vi "cubeSubstraction.vi"() -> ()   [LabVIEW 2016]
panel:
  out "size(s) 3":i32[](array[numeric])
  out "processed cube 2":i32[][](graph)
  out "reference":i32[][](graph)
  out "processed cube":i32[][](graph)
  out "raw cube":i32[][](graph)
  out "size(s)":i32[](array[numeric])
  out "size(s) 2":i32[](array[numeric])
  out "x-y":i32[][][](array[numeric])
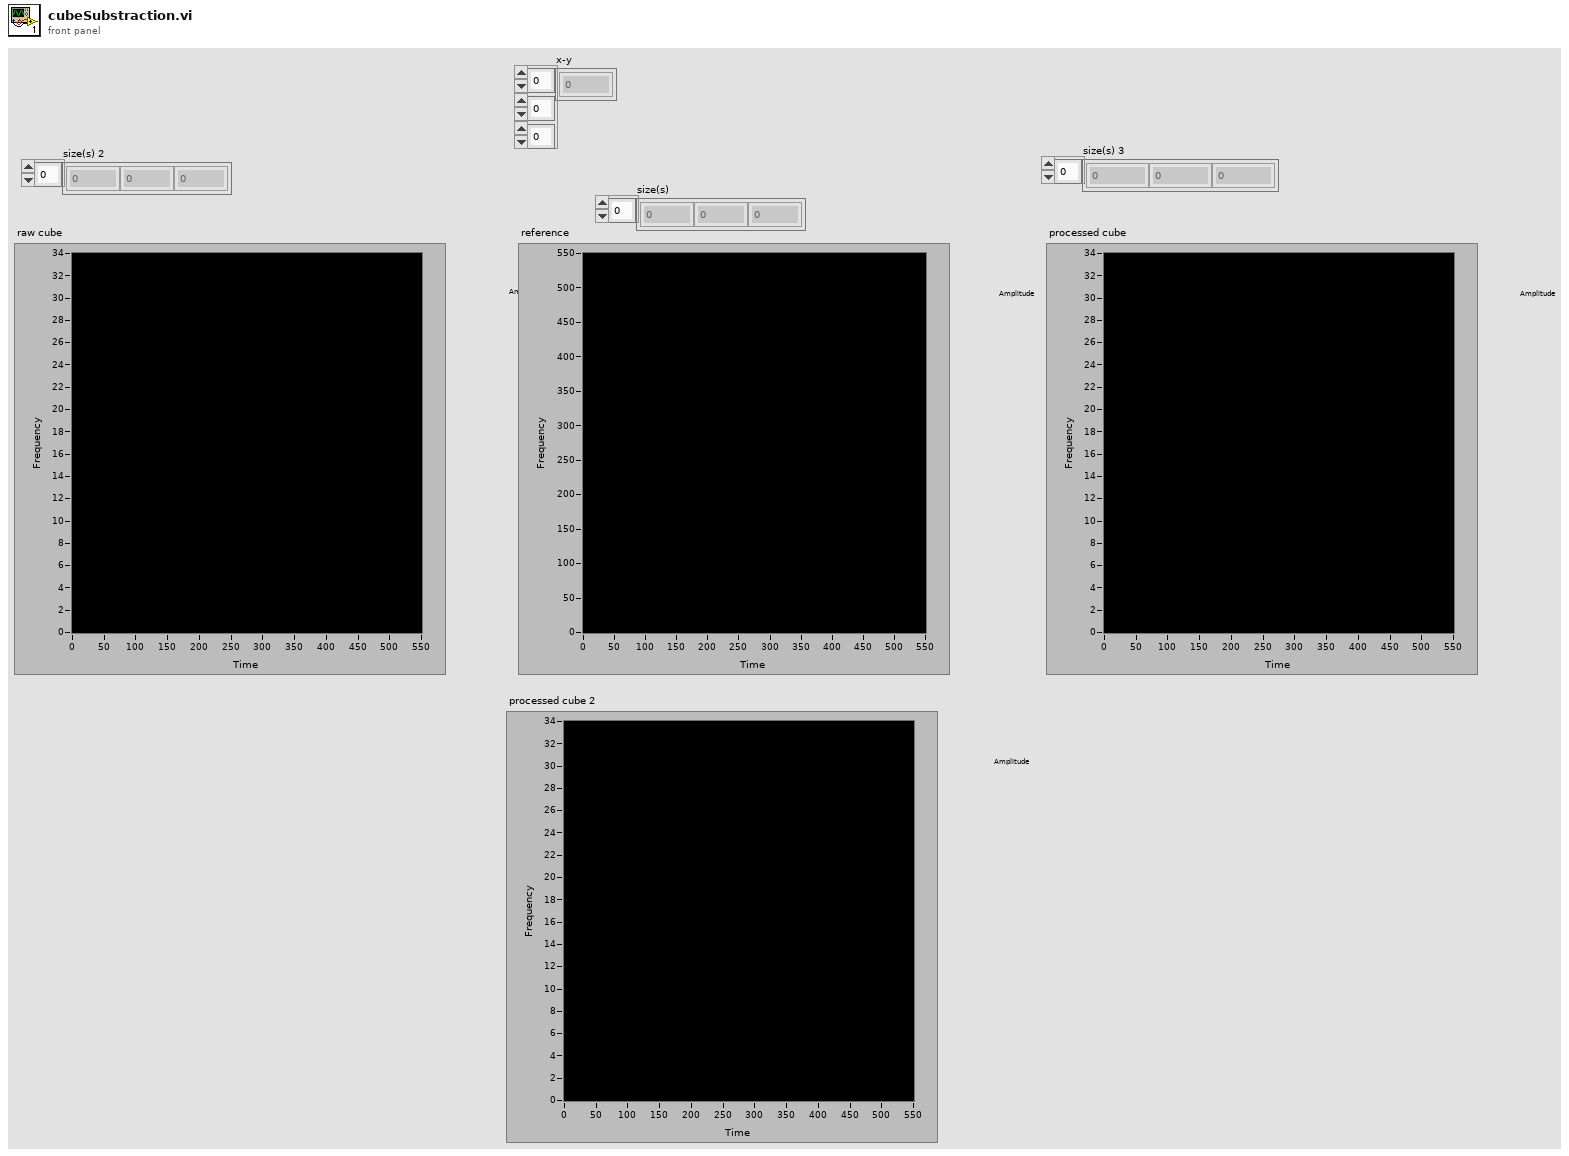
[diagram p1: front panel]
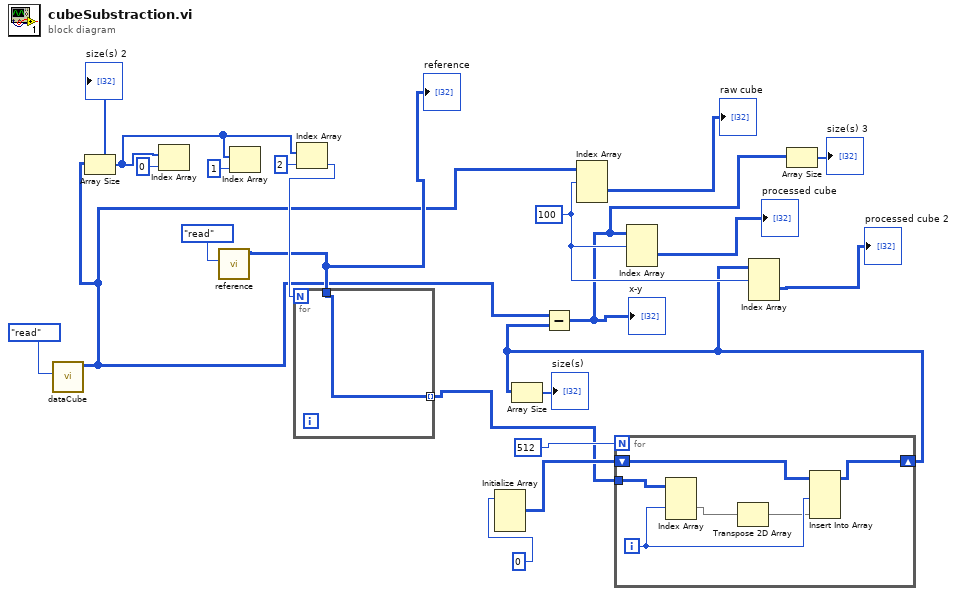
[diagram p0: block diagram]
diagram:
  w7 = 100 ("index")
  n1 = call "dataCube.vi"("Enum"=enum16{"clear", "read", "write"}."read") -> ("imageCubeOut"=w1:i32[][][])  [unwired: 8 in, 2 out]
  n2 = Array Size(array=w1) -> (size(s)=w20:i32[])
  "size(s) 2" <- w20
  n3 = Index Array(array=w20, index=0) -> ()  [unwired: 1 out]
  n4 = call "reference.vi"("Enum"=enum16{"clear", "read", "write"}."read") -> ("referenceImageOut"=w9:i32[][])  [unwired: 10 in]
  "reference" <- w9
  n5 = Index Array(array=w20, index=1) -> ()  [unwired: 1 out]
  n6 = Index Array(array=w20, index=2) -> (element=w16:i32)
  n7 = for {
    N: w16 -> [_]
    tunnel: w9 -> [w22]
    tunnel: [w22] -> w8 mode=indexing
  }
  n8 = Initialize Array(0 ("element")) -> (w11:i32[][][])  [unwired: 3 in]
  n9 = Index Array(array=w1, index (dim 0)=w7) -> (element=→"raw cube":i32[][])  [unwired: 2 in]
  n10 = for {
    N: 512 -> [_]
    tunnel: w8 -> [w28]
    shift-right: [w26] -> w2
    shift-left: w11 -> [w25]
    i -> [w24]
    n11 = Index Array(array=w28, index (dim 1)=w24) -> (element=w27:i32[][])  [unwired: 2 in]
    n12 = Transpose 2D Array(2D array=w27) -> (transposed array=w23:i32[][])
    n13 = Insert Into Array(array=w25, index (dim 1)=w24, new element=w23) -> (w26:i32[][][])  [unwired: 2 in]
  }
  n14 = Array Size(array=w2) -> (size(s)=→"size(s)":i32[])
  n15 = Subtract(x=w1, y=w2) -> (x-y=w3:i32[][][])
  "x-y" <- w3
  n16 = Index Array(array=w3, index (dim 0)=w7) -> (element=→"processed cube":i32[][])  [unwired: 2 in]
  n17 = Index Array(array=w2, index (dim 0)=w7) -> (element=→"processed cube 2":i32[][])  [unwired: 2 in]
  n18 = Array Size(array=w3) -> (size(s)=→"size(s) 3":i32[])
